vi "Mouse Move Event.vi"(8 "error in":errorcluster, 9 "Position":cluster{"dx":u32, "dy":u32}) -> (0 "error out":errorcluster)   [LabVIEW 2012]
uses:
  C:/Windows/System32/user32.dll
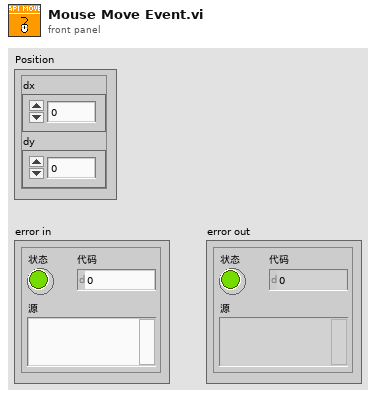
[diagram p1: front panel]
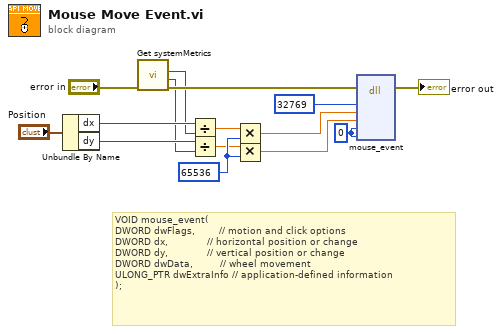
[diagram p0: block diagram]
diagram:
  w6 = u32 65536 ("y")
  w15 = u32 0 ("dwExtraInfo")
  # "VOID mouse_event(\nDWORD dwFlags,        // motion and click options\nDWORD dx,             // horizontal position or change\nDWORD dy,             // vertical position or change\nDWORD dwData,         // wheel movement\nULONG_PTR dwExtraInfo // application-defined information\n);"
  n1 = Unbundle By Name("Position") -> ("dx"=w8:u32, "dy"=w7:u32)
  n2 = call "Get systemMetrics.vi"("error in"="error in") -> ("error out"=w12:errorcluster, "height"=w2:u32, "width"=w3:u32)  [unwired: 8 in]
  n3 = Divide(x=w8, y=w3) -> (x/y=w4:dbl)
  n4 = Divide(x=w7, y=w2) -> (x/y=w5:dbl)
  n5 = Multiply(x=w4, y=w6) -> (x*y=w11:dbl)
  n6 = Multiply(x=w5, y=w6) -> (x*y=w10:dbl)
  n7 = dll-call lib="C:/Windows/System32/user32.dll" fn="mouse_event"(error in=w12, "dwFlags"=u32 32769, "dx"=w11, "dy"=w10, "dwData"=w15, "dwExtraInfo"=w15) -> (error out=→"error out":errorcluster)  [unwired: 8 in, 1 out]
